vi "MenuSelect.vi"(8 "error in":errorcluster caption="错误输入（无错误）", 10 "Tag":string, 11 "PanelRootNode 输入":refnum<class "PanelRootNode.lvclass"> caption="DNL_LabVIEW Object in") -> (0 "error out":errorcluster caption="错误输出", 3 "PanelRootNode 输出":refnum<class "PanelRootNode.lvclass"> caption="DNL_LabVIEW Object out")   [LabVIEW 2016, in "PanelRootNode.lvclass"]
uses:
  PanelRootNode.lvclass
  PanelDataNode/Split Mode.ctl
  PanelDataNode/PanelDataNode.lvclass
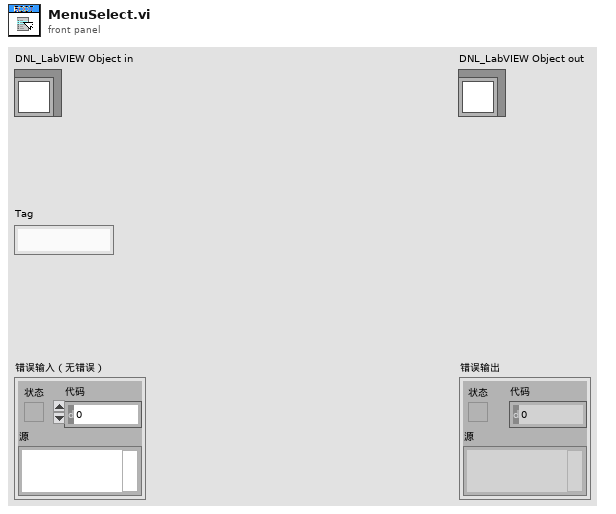
[diagram p1: front panel]
types:
  T1 = typedef "PanelDataNode.lvclass/Split Mode.ctl" = enum16{"Horizontal(up)", "Vertical(left)", "Horizontal(down)", "Vertical(right)"}
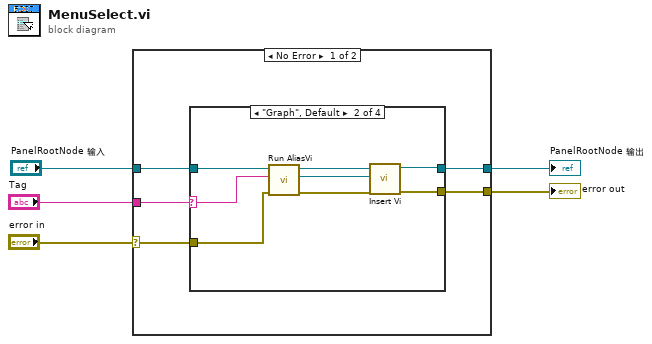
[diagram p0: block diagram]
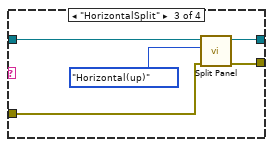
[diagram p3: hidden frame]
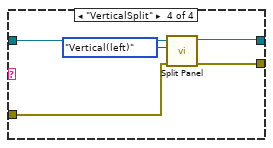
[diagram p4: hidden frame]
diagram:
  n1 = case shown="No Error" "error in" {
    selector: "error in" -> [w6 w32]
    tunnel: [w7 w32] -> w4
    tunnel: [w9 w31] -> w2
    tunnel: "PanelRootNode 输入" -> [w10 w31]
    tunnel: "Tag" -> [w8 _]
    frame No Error {
      n2 = case shown="\"Graph\", Default" w8 {
        selector: w8 -> [_ w15 _ _]
        tunnel: w10 -> [w12 w20 w25 w30]
        tunnel: [w12 w18 w24 w29] -> w9
        tunnel: [w11 w14 w22 w27] -> w7
        tunnel: w6 -> [w11 w13 w21 w26]
        frame "" {
        }
        frame "Graph", Default {
          n3 = call-dynamic "Run AliasVi.vi"("error in (no error)"=w13, "Vi Alias"=w15, "PanelDataNode 输入"=w20) -> ("error out"=w16:errorcluster, "VI*"=w17:refnum<vi>, "PanelDataNode 输出"=w19:refnum<class "PanelRootNode.lvclass">)  [unwired: 6 in]
          n4 = call-dynamic "Insert Vi.vi"("error in (no error)"=w16, "VI*"=w17, "PanelDataNode 输入"=w19) -> ("error out"=w14:errorcluster, "PanelDataNode 输出"=w18:refnum<class "PanelRootNode.lvclass">)  [unwired: 7 in]
        }
        frame "HorizontalSplit" {
          n5 = call-dynamic "Split Panel.vi"("error in"=w21, "Split Mode"=Split_Mode."Horizontal(up)", "PanelDataNode 输入"=w25) -> ("error out"=w22:errorcluster, "PanelDataNode 输出"=w24:refnum<class "PanelRootNode.lvclass">)  [unwired: 6 in, 1 out]
        }
        frame "VerticalSplit" {
          n6 = call-dynamic "Split Panel.vi"("error in"=w26, "Split Mode"=Split_Mode."Vertical(left)", "PanelDataNode 输入"=w30) -> ("error out"=w27:errorcluster, "PanelDataNode 输出"=w29:refnum<class "PanelRootNode.lvclass">)  [unwired: 6 in, 1 out]
        }
      }
    }
    frame Error {
    }
  }
  "error out" <- w4
  "PanelRootNode 输出" <- w2
